vi "Draw Robot.vi"(9 "Picture  Reference":refnum<vi>, 10 "Pose":cluster{"x":dbl, "y":dbl, "theta":dbl}, 11 "Picture In":picture) -> (3 "Picture Out":picture)   [LabVIEW 2020]
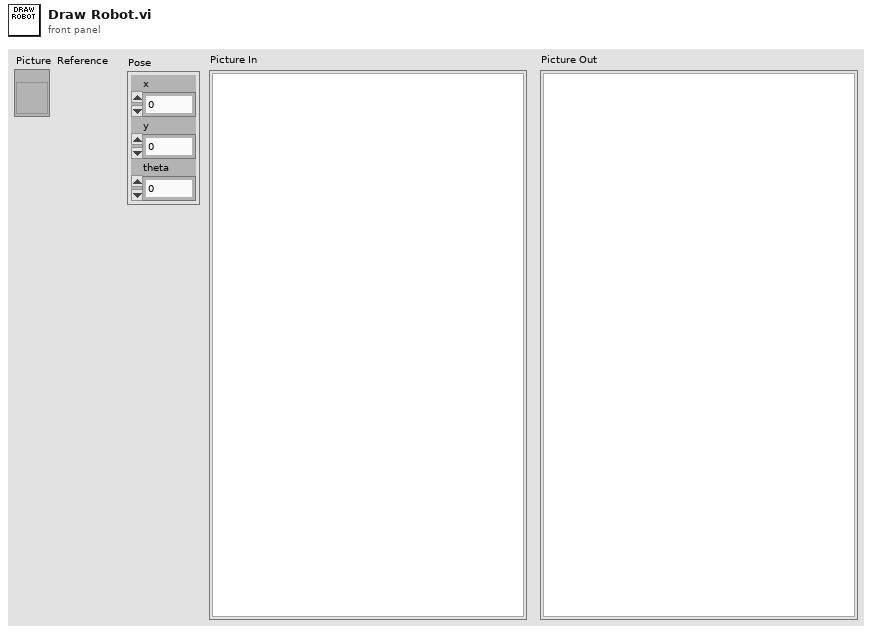
[diagram p1: front panel]
types:
  T1 = typedef "LVBoundsTypeDef.ctl" = cluster{"Width":u32, "Height":u32}
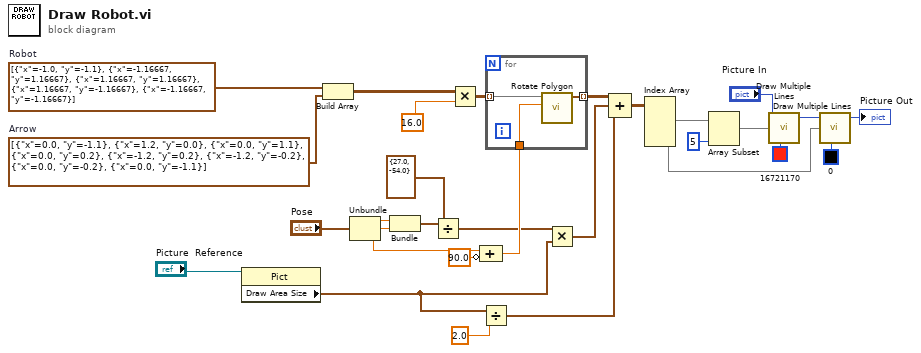
[diagram p0: block diagram]
diagram:
  w27 = cluster{"x":dbl, "y":dbl}[] [{"x"=-1.0, "y"=-1.1}, {"x"=-1.16667, "y"=1.16667}, {"x"=1.16667, "y"=1.16667}, {"x"=1.16667, "y"=-1.16667}, {"x"=-1.16667, "y"=-1.16667}]  # Robot
  w26 = cluster{"x":dbl, "y":dbl}[] [{"x"=0.0, "y"=-1.1}, {"x"=1.2, "y"=0.0}, {"x"=0.0, "y"=1.1}, {"x"=0.0, "y"=0.2}, {"x"=-1.2, "y"=0.2}, {"x"=-1.2, "y"=-0.2}, {"x"=0.0, "y"=-0.2}, {"x"=0.0, "y"=-1.1}]  # Arrow
  n1 = property class="Pict"(reference="Picture  Reference") -> ("Draw Area Size"=w1:T1)  [unwired: 1 in, 2 out]
  n2 = Build Array(w27, w26) -> (w25:cluster{"x":dbl, "y":dbl}[][])
  n3 = Unbundle("Pose") -> ("x"=w19:dbl, "y"=w18:dbl, "theta"=w20:dbl)
  n4 = Bundle("x"=w19, "y"=w18) -> (w12:cluster{"x":dbl, "y":dbl})  [unwired: 1 in]
  n5 = Divide(x=w12, y=cluster{"x":dbl, "y":dbl} {"x"=27.0, "y"=-54.0}) -> (x/y=w10:cluster{"x":dbl, "y":dbl})
  n6 = Multiply(x=w25, y=16.0 ("Scale")) -> (x*y=w29:cluster{"x":dbl, "y":dbl}[][])
  n7 = Compound Arithmetic op=ADD(w20, invert 90.0 ("value")) -> (w21:dbl)
  n8 = Divide(x=w1, y=2.0) -> (x/y=w14:cluster{"Width":dbl, "Height":dbl})
  n9 = for {
    tunnel: w21 -> [w31]
    tunnel: [w32] -> w16 mode=indexing
    tunnel: w29 -> [w33] mode=indexing
    n10 = call "Rotate Polygon.vi"("Angle"=w31, "Input Polygon"=w33) -> ("Output Polygon"=w32:cluster{dbl, dbl}[])  [unwired: 9 in]
  }
  n11 = Multiply(x=w10, y=w1) -> (x*y=w9:cluster{dbl, dbl})
  n12 = Compound Arithmetic op=ADD(w16, w9, w14) -> (w15:cluster{dbl, dbl}[][])
  n13 = Index Array(array=w15) -> (element #1=w6:cluster{dbl, dbl}[], element #2=w23:cluster{dbl, dbl}[])  [unwired: 4 in]
  n14 = Array Subset(array=w6, length=5) -> (w5:cluster{dbl, dbl}[])  [unwired: 1 in]
  n15 = call <vilib>:"Draw Multiple Lines.vi"("picture"="Picture In", "line endpoints"=w5, "color(black)"=u32 16721170) -> ("new picture"=w22:picture)  [unwired: 6 in]
  n16 = call <vilib>:"Draw Multiple Lines.vi"("picture"=w22, "line endpoints"=w23, "color(black)"=u32 0) -> ("new picture"=→"Picture Out":picture)  [unwired: 6 in]
